vi "Query - String - 2D.vi"(8 "error in":errorcluster, 10 "Query":string, 11 "Module ID":i32=-1) -> (0 "error out":errorcluster, 1 "Meta Data":variant, 2 "Return Data":string[][](array[string]), 4 "Field Names":string[](array[string]))   [LabVIEW 2014, in "DB_CONNECTOR.lvlib"]
uses:
  DB_CONNECTOR.lvlib
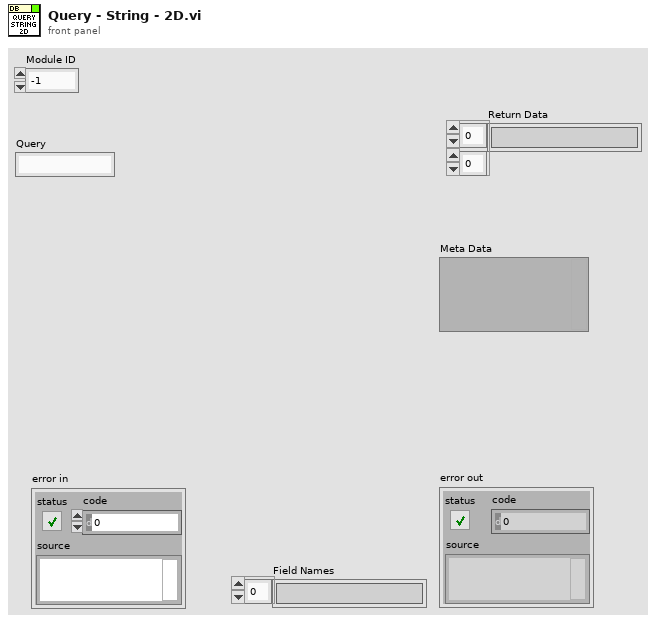
[diagram p1: front panel]
types:
  T1 = typedef "DB_CONNECTOR.lvlib/Query (Reply Payload)--cluster.ctl" = cluster{"Return Data":string[][], "Meta Data":variant, "Field Names":string[], "Query_error":errorcluster}
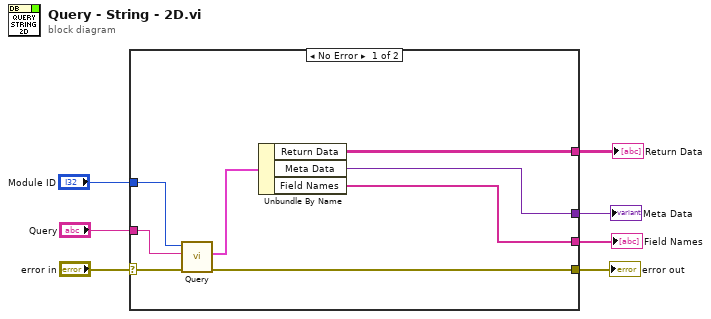
[diagram p0: block diagram]
diagram:
  n1 = case shown="No Error" "error in" {
    selector: "error in" -> [w15 w16]
    tunnel: [w10 w16] -> w6
    tunnel: "Query" -> [w13 _]
    tunnel: "Module ID" -> [w12 _]
    tunnel: [w11 _] -> w3
    tunnel: [w9 _] -> w2
    tunnel: [w8 _] -> w1
    frame No Error {
      n2 = call "Query.vi"("error in (no error)"=w15, "Query"=w13, "Module ID"=w12) -> ("error out"=w10:errorcluster, "Reply Payload"=w14:T1)  [unwired: 7 in]
      n3 = Unbundle By Name(w14) -> ("Return Data"=w11:string[][], "Meta Data"=w9:variant, "Field Names"=w8:string[])
    }
    frame Error {
    }
  }
  "error out" <- w6
  "Return Data" <- w3
  "Meta Data" <- w2
  "Field Names" <- w1
